vi "Intake Brain.vi"(6 "Floor_Pickup":bool, 9 "Ele_At_Pos":bool, 10 "Floor_Pickup_High":bool, 11 "Tote_Sensor_1":bool) -> (1 "Exit_Auto":bool, 2 "Store_Auto":bool, 3 "Store_Auto_High":bool, 4 "Infeed cmd":dbl)   [LabVIEW 2014]
uses:
  General_VI/Global Var.vi
panel:
  out "Auto_State":i32(graph)
  out "State":i32
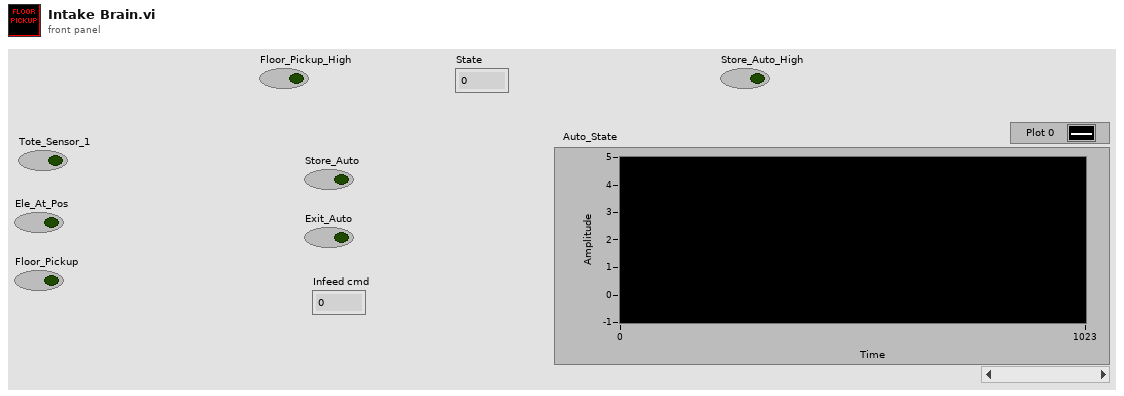
[diagram p1: front panel]
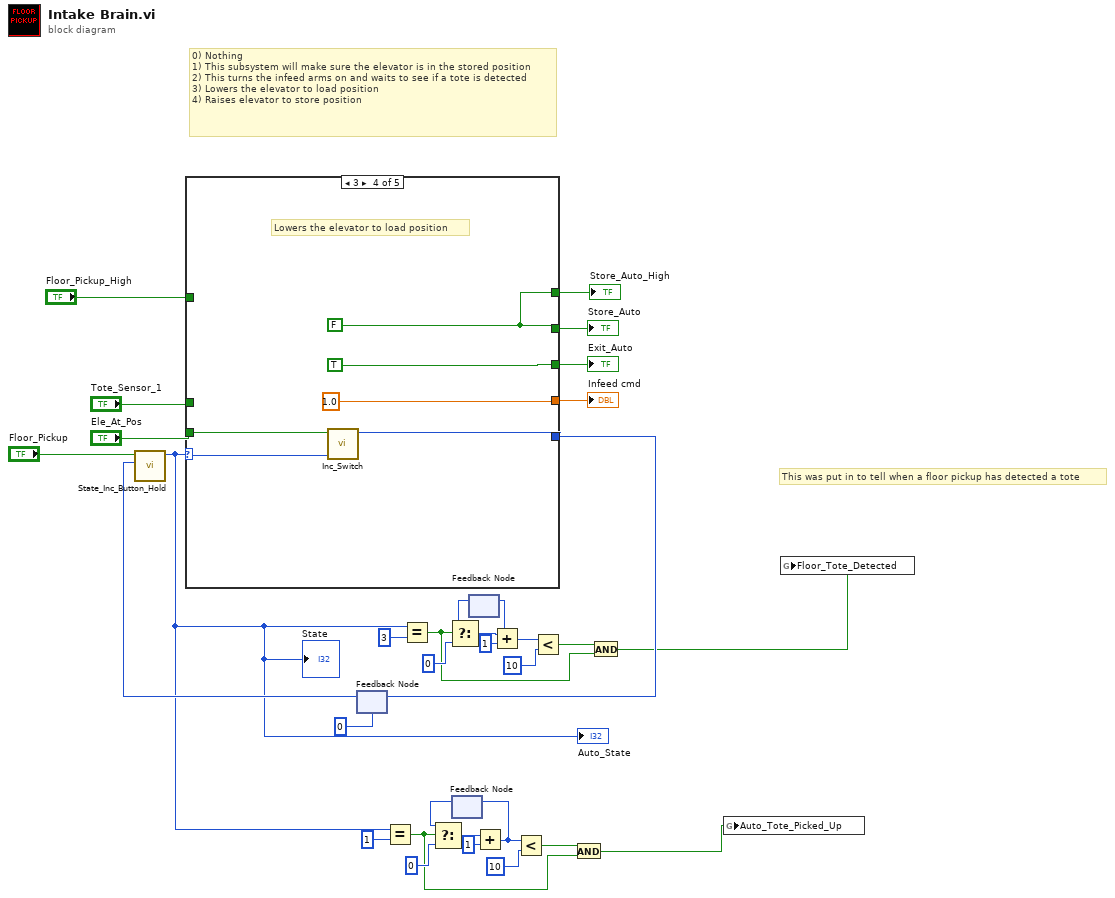
[diagram p0: block diagram]
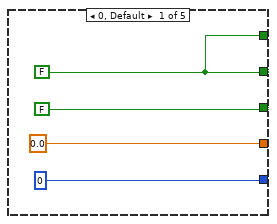
[diagram p2: hidden frame]
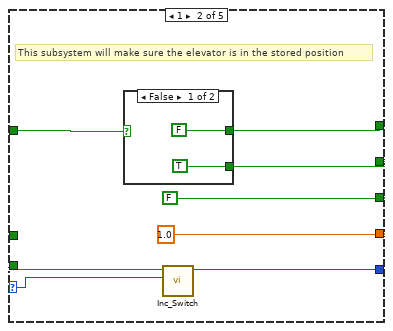
[diagram p3: hidden frame]
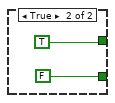
[diagram p4: hidden frame]
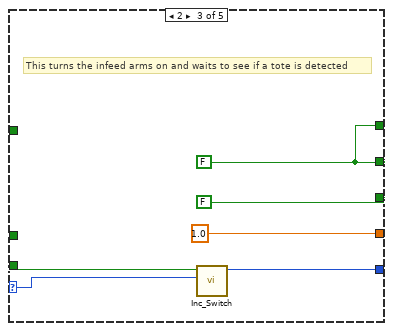
[diagram p5: hidden frame]
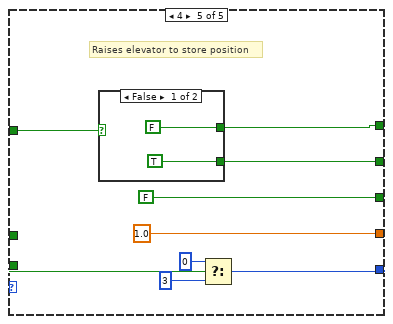
[diagram p6: hidden frame]
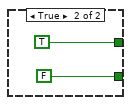
[diagram p7: hidden frame]
diagram:
  # "This was put in to tell when a floor pickup has detected a tote"
  # "0) Nothing\n1) This subsystem will make sure the elevator is in the stored position\n2) This turns the infeed arms on and waits to see if a tote is detected \n3) Lowers the elevator to load position \n4) Raises elevator to store position"
  n1 = feedback #1(0 ("Numeric out")) -> (w26:i32)
  n2 = call "State_Inc_Button_Hold.vi"("Numeric in"=w26, "Floor_Pickup"="Floor_Pickup") -> ("t"=w7:i32)  [unwired: 9 in]
  "State" <- w7
  "Auto_State" <- w7
  n3 = case shown="3" w7 {
    selector: w7 -> [_ w39 w52 w56 _]
    tunnel: "Tote_Sensor_1" -> [_ _ w51 _ _]
    tunnel: "Ele_At_Pos" -> [_ w41 _ w58 w66]
    tunnel: [w33 w43 w49 w55 w69] -> w30
    tunnel: [FALSE FALSE FALSE TRUE FALSE] -> w31
    tunnel: [0 w40 w50 w57 w65] -> w24
    tunnel: [0.0 1.0 1.0 ("f") 1.0 1.0] -> w32
    tunnel: [w33 w37 w49 w55 w62] -> w2
    tunnel: "Floor_Pickup_High" -> [_ w38 _ _ w61]
    frame 0, Default {
      w33 = FALSE
    }
    frame 1 {
      # "This subsystem will make sure the elevator is in the stored position"
      n4 = case shown="False" w38 {
        tunnel: [TRUE FALSE] -> w43
        tunnel: [FALSE TRUE] -> w37
        frame False {
        }
        frame True {
        }
      }
      n5 = call "Inc_Switch.vi"("Numeric in"=w39, "Ele_At_Pos"=w41) -> ("Numeric out"=w40:i32)  [unwired: 9 in]
    }
    frame 2 {
      w49 = FALSE
      # "This turns the infeed arms on and waits to see if a tote is detected"
      n6 = call "Inc_Switch.vi"("Numeric in"=w52, "Ele_At_Pos"=w51) -> ("Numeric out"=w50:i32)  [unwired: 9 in]
    }
    frame 3 {
      w55 = FALSE
      # "Lowers the elevator to load position"
      n7 = call "Inc_Switch.vi"("Numeric in"=w56, "Ele_At_Pos"=w58) -> ("Numeric out"=w57:i32)  [unwired: 9 in]
    }
    frame 4 {
      # "Raises elevator to store position"
      n8 = case shown="False" w61 {
        tunnel: [TRUE FALSE] -> w69
        tunnel: [FALSE TRUE] -> w62
        frame False {
        }
        frame True {
        }
      }
      n9 = Select(t=0, s=w66, f=3) -> (s? t:f=w65:i32)
    }
  }
  "Infeed cmd" <- w32
  "Exit_Auto" <- w31
  "Store_Auto" <- w30
  "Store_Auto_High" <- w2
  n10 = feedback-in #1(w24) -> ()
  n11 = Equal?(x=w7, y=1) -> (x = y?=w6:bool)
  n12 = Equal?(x=w7, y=3) -> (x = y?=w15:bool)
  n13 = feedback #2() -> (w5:i32)  [unwired: 1 in]
  n14 = Select(t=w5, s=w6, f=0) -> (s? t:f=w11:i32)
  n15 = feedback #3() -> (w19:i32)  [unwired: 1 in]
  n16 = Select(t=w19, s=w15, f=0) -> (s? t:f=w21:i32)
  n17 = Add(x=w11, y=1) -> (x+y=w3:i32)
  n18 = feedback-in #2(w3) -> ()
  n19 = Add(x=w21, y=1) -> (x+y=w18:i32)
  n20 = feedback-in #3(w18) -> ()
  n21 = Less?(x=w3, y=10) -> (x < y?=w8:bool)
  n22 = Less?(x=w18, y=10) -> (x < y?=w16:bool)
  n23 = And(x=w8, y=w6) -> (x .and. y?=w4:bool)
  n24 = And(x=w16, y=w15) -> (x .and. y?=w14:bool)
  n25 = global write "Global Var.vi" "Auto_Tote_Picked_Up"(w4) -> ()
  n26 = global write "Global Var.vi" "Floor_Tote_Detected"(w14) -> ()
